vi "SetConfiguration.vi"(8 "error in (no error)":errorcluster, 10 "Configuration":variant, 11 "Measurement in":refnum<class "Measurement.lvclass">) -> (0 "error out":errorcluster, 3 "Measurement out":refnum<class "Measurement.lvclass">)   [LabVIEW 2019, in "Measurement.lvclass"]
uses:
  Measurement.lvclass
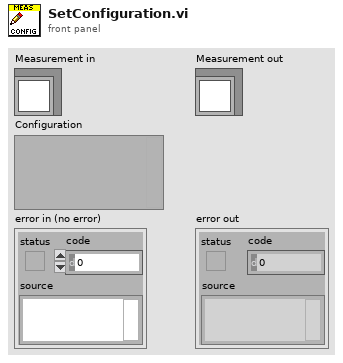
[diagram p1: front panel]
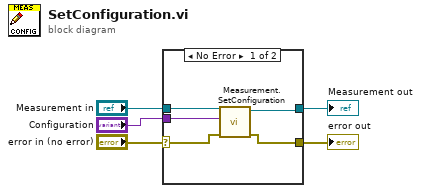
[diagram p0: block diagram]
diagram:
  n1 = case shown="No Error" "error in (no error)" {
    selector: "error in (no error)" -> [w8 w12]
    tunnel: [w6 w12] -> w4
    tunnel: [w7 w11] -> w2
    tunnel: "Measurement in" -> [w10 w11]
    tunnel: "Configuration" -> [w9 _]
    frame No Error {
      n2 = call-dynamic "Measurement.SetConfiguration.vi"("error in (no error)"=w8, "Configuration"=w9, "Measurement in"=w10) -> ("error out"=w6:errorcluster, "Measurement out"=w7:refnum<class "Measurement.lvclass">)  [unwired: 7 in]
    }
    frame Error {
    }
  }
  "error out" <- w4
  "Measurement out" <- w2
